vi "Mask ROI FG.vi"(8 "error in (no error)":errorcluster, 10 "Mask ROI In":T2={"left annulus"={"Center X"=929, "Center Y"=663, "Inner Radius"=200, "Outer Radius"=405, "Start Angle"=90.0, "End Angle"=180.0}, "right annulus"={"Center X"=929, "Center Y"=663, "Inner Radius"=200, "Outer Radius"=405, "Start Angle"=90.0, "End Angle"=180.0}, "Threshold Range"={"Lower value"=106.82432432432432, "Upper value"=255.0}, "[Avg BG]"=[], "Number of Sectors"=0, "Left ROI"={"Global Rectangle"=[], "Contours"=[]}, "Right ROI"={"Global Rectangle"=[], "Contours"=[]}} {"Right ROI"."Contours"."Type" items=["No Selection", "Point", "Line", "Rectangle", "Oval", "Polygon", "Freehand Region", "Annulus", "Unused2", "Unused3", "Broken Line", "Freehand Line", "Rotated Rectangle"]; "Left ROI"."Contours"."Type" items=["No Selection", "Point", "Line", "Rectangle", "Oval", "Polygon", "Freehand Region", "Annulus", "Unused2", "Unused3", "Broken Line", "Freehand Line", "Rotated Rectangle"]; "Threshold Range"."Upper value" min=0.0 max=255.0 scale=0.0..255.0; "Threshold Range"."Lower value" min=0.0 max=255.0 scale=0.0..255.0; "right annulus"."End Angle" format="%.2f"; "right annulus"."Start Angle" format="%.2f"; "right annulus"."Center X" scale=0.0..1024.0; "left annulus"."End Angle" format="%.2f"; "left annulus"."Start Angle" format="%.2f"; "left annulus"."Center X" scale=0.0..1024.0}, 11 "Operation":T1) -> (0 "error out":errorcluster, 2 "Mask ROI Out":T2={"left annulus"={"Center X"=929, "Center Y"=663, "Inner Radius"=200, "Outer Radius"=405, "Start Angle"=90.0, "End Angle"=180.0}, "right annulus"={"Center X"=929, "Center Y"=663, "Inner Radius"=200, "Outer Radius"=405, "Start Angle"=90.0, "End Angle"=180.0}, "Threshold Range"={"Lower value"=106.82432432432432, "Upper value"=255.0}, "[Avg BG]"=[], "Number of Sectors"=0, "Left ROI"={"Global Rectangle"=[], "Contours"=[]}, "Right ROI"={"Global Rectangle"=[], "Contours"=[]}} {"Right ROI"."Contours"."Type" items=["No Selection", "Point", "Line", "Rectangle", "Oval", "Polygon", "Freehand Region", "Annulus", "Unused2", "Unused3", "Broken Line", "Freehand Line", "Rotated Rectangle"]; "Left ROI"."Contours"."Type" items=["No Selection", "Point", "Line", "Rectangle", "Oval", "Polygon", "Freehand Region", "Annulus", "Unused2", "Unused3", "Broken Line", "Freehand Line", "Rotated Rectangle"]; "Threshold Range"."Upper value" min=0.0 max=255.0 scale=0.0..255.0; "Threshold Range"."Lower value" min=0.0 max=255.0 scale=0.0..255.0; "right annulus"."End Angle" format="%.2f"; "right annulus"."Start Angle" format="%.2f"; "right annulus"."Center X" scale=0.0..1024.0; "left annulus"."End Angle" format="%.2f"; "left annulus"."Start Angle" format="%.2f"; "left annulus"."Center X" scale=0.0..1024.0})   [LabVIEW 2013]
uses:
  Mask ROI Cluster.ctl
  Mask ROI FG Enum.ctl
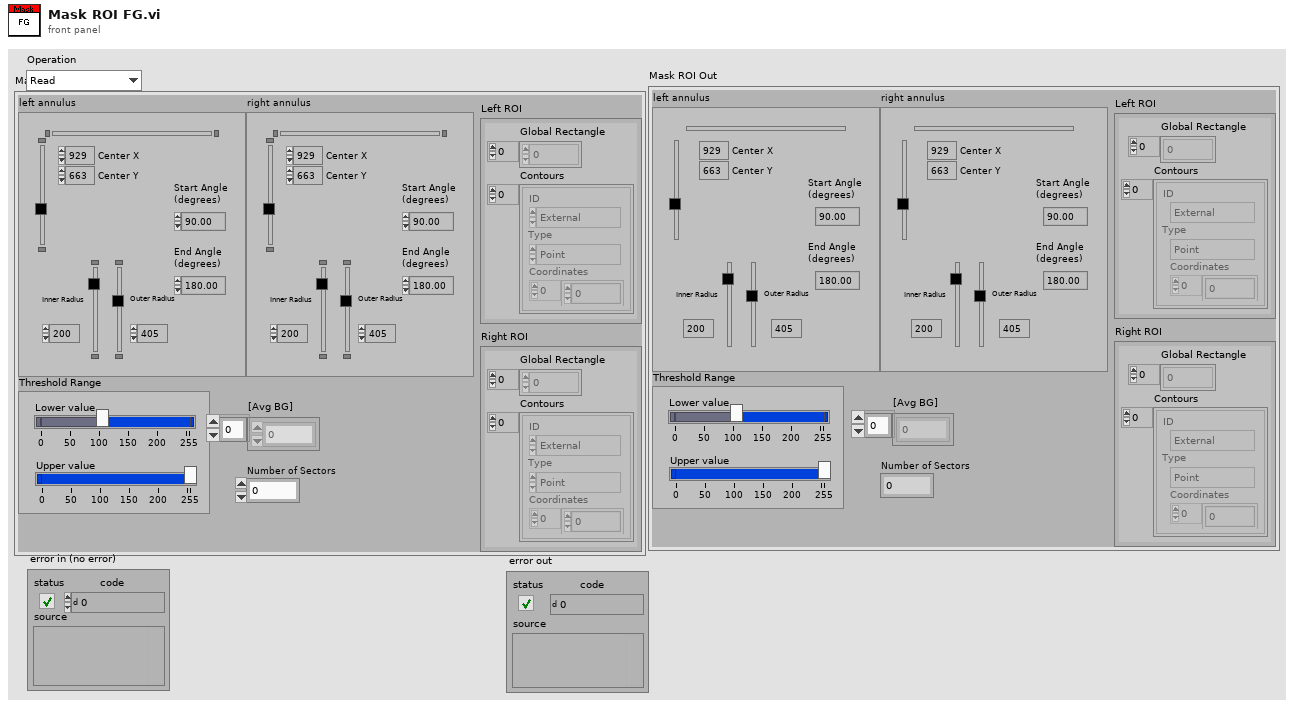
[diagram p1: front panel]
types:
  T1 = typedef "Mask ROI FG Enum.ctl" = enum16{"Read", "Write"}
  T2 = typedef "Mask ROI Cluster.ctl" = cluster{"left annulus":T3, "right annulus":T3, "Threshold Range":cluster{"Lower value":dbl, "Upper value":dbl}, "[Avg BG]":u8[], "Number of Sectors":u8, "Left ROI":T4, "Right ROI":T4}
  T3 = typedef "IMAQ Circle" = cluster{"Center X":i32, "Center Y":i32, "Inner Radius":i32, "Outer Radius":i32, "Start Angle":dbl, "End Angle":dbl}
  T4 = typedef "ROI Descriptor" = cluster{"Global Rectangle":i32[], "Contours":cluster{"ID":enum32{"External", "Internal"}, "Type":u32, "Coordinates":i32[]}[]}
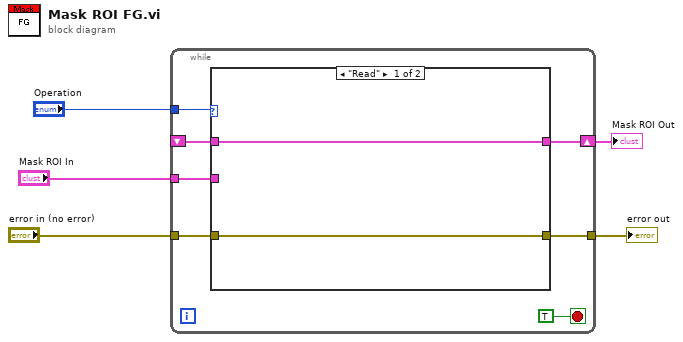
[diagram p0: block diagram]
diagram:
  n1 = while {
    tunnel: "Operation" -> [w11]
    tunnel: "Mask ROI In" -> [w10]
    shift-right: [w9] -> w3
    shift-left: _ -> [w8]
    tunnel: [w7] -> w2
    tunnel: "error in (no error)" -> [w6]
    stop <- TRUE stop-if-true
    n2 = case shown="\"Read\"" w11 {
      tunnel: w10 -> [_ w16]
      tunnel: [w14 w16] -> w9
      tunnel: w8 -> [w14 _]
      tunnel: [w13 w15] -> w7
      tunnel: w6 -> [w13 w15]
      frame "Read" {
      }
      frame "Write" {
      }
    }
  }
  "Mask ROI Out" <- w3
  "error out" <- w2
